vi "initialize daq.vi"(6 "input limits (no change)":cluster{"high limit":sgl, "low limit":sgl}[](array[cluster]) {"low limit" format="%.2f"; "high limit" format="%.2f"}, 7 "taskID in":u32 format="%.0x", 8 "buffer size\n(4000 scans)":i32=400, 9 "interchannel delay\nin secs ( -1: hw default)":sgl=-1.0 format="%.2p", 10 "channels (0)":string[](array[string])=["ob0 ! sc1 ! md1 ! 0:31", "ob0 ! sc1 ! md2 ! 0:31"], 11 "device (1)":i16=1) -> (0 "error out":errorcluster={"status"=TRUE, "code"=-10001, "source"="AI Group Config"}, 1 "group channel settings":T1(array[cluster]) {"scale offset" format="%.2f"; "scale multiplier" format="%.5e"; "gain" format="%.2f"; "range" format="%.2f"; "lower input limits" format="%.2f"; "upper input limits" format="%.2f"}, 3 "taskID out":u32 format="%.0x")   [LabVIEW 2010]
doc: "Cont(inuous) Acq(uire) & Chart (buffered) demonstrates buffered data acquisition. Data is continuously acquired into a circular buffer at the same time that data previously retrieved from the buffer is plotted. This VI also demonstrates how to plot multiple points from multiple channels on a chart. \n\nBefore running this VI, set the values of the controls on the front panel. Select Show Help Window from the Help menu to see a description of each control. If the values you select for all the controls are values you will usually use, select Make Current Values Default from the Operate menu and save the VI. Or, you may save individual control's default values by popping up on the control, selecting Data Operations, then selecting Make Current Value Default, and saving the VI.\n\n\nThe buffer size is the number of scans that will be held in the internal memory buffer, and is limited by the amount of memory available. In order to keep up with the scan rate as best as possible, this VI retrieves either \"min # of scans to read at a time\" or the scan backlog from the previous AI Read call, whichever is greater. Experiment with the buffer size and the number of scans to read each time. If the buffer is too small or you are not reading data from it fast enough, your data will be overwritten by new data before you have a chance to read it (overwrite error). If the buffer is too big, you will run out of memory (out of memory error).\n\n\nYou will probably want to add more functions to the diagram to customize this VI for your application. A common reason to read data while the acquisition is in progress is to process and display the data in pseudo-real time. The acquisition rate you can achieve depends on how much processing and display the VI must do. This VI calls a subVI named My Data Processing. Add whatever processing you need to this subVI, or replace it with one of your own. The data processing subVI also demonstrates how to use error clusters in your own subVIs, so they can be included in the error data flow chain. Note that the amount of the data returned will change depending on the scan backlog. Use the \"number read\" output from the AI Read VI to determine how many scans are returned."
panel:
  # "For instructions\nselect Show VI Info\nfrom the Windows menu."
  # "hardware settings"
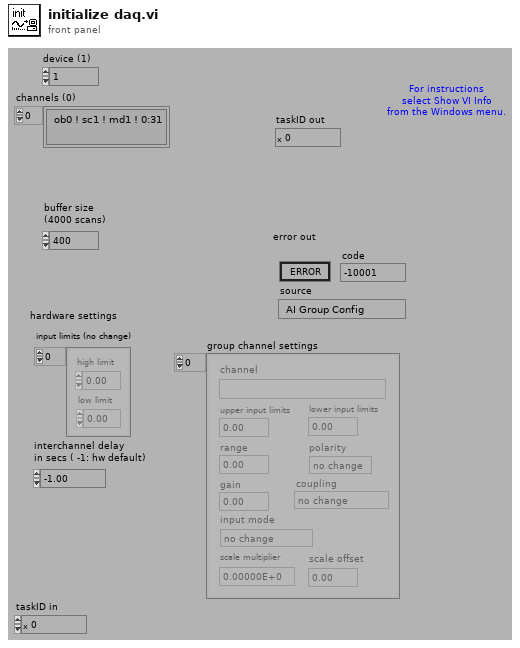
[diagram p1: front panel]
types:
  T1 = cluster{"channel":string, "upper input limits":sgl, "lower input limits":sgl, "range":sgl, "polarity":enum16{"no change", "bipolar", "unipolar"}, "gain":sgl, "coupling":enum16{"no change", "DC", "AC", "ground", "internal reference"}, "input mode":enum16{"no change", "differential", "rse", "nrse"}, "scale multiplier":sgl, "scale offset":sgl}[]
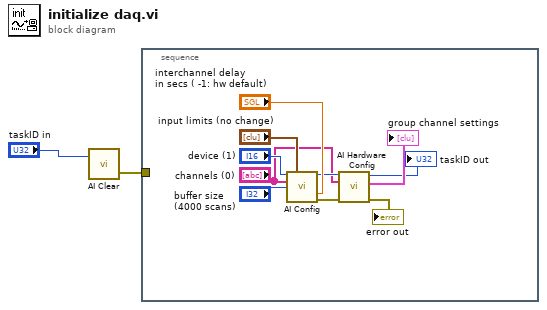
[diagram p0: block diagram]
diagram:
  n1 = call <vilib>:"AI Clear.vi"("taskID in"="taskID in") -> ("error out"=w2:errorcluster)  [unwired: 5 in, 1 out]
  n2 = stacked-sequence {
    tunnel: w2 -> [_]
    frame #0 {
      n3 = call <vilib>:"AI Config.vi"("device (1)"="device (1)", "input limits (no change)"="input limits (no change)", "channels (0)"="channels (0)", "buffer size (1000 scans)"="buffer size\n(4000 scans)", "interchannel delay (secs) (board default)"="interchannel delay\nin secs ( -1: hw default)") -> ("taskID"=w6:u32, "error out"=w7:errorcluster)  [unwired: 8 in, 1 out]
      n4 = call <vilib>:"AI Hardware Config.vi"("error in (no error)"=w7, "channel list (empty)"="channels (0)", "task ID"=w6) -> ("error out"=→"error out":errorcluster, "group channel settings"=→"group channel settings":T1, "task ID out"=→"taskID out":u32)  [unwired: 6 in]
    }
  }
